vi "wformFileRead.vi"() -> ()   [LabVIEW 2014]
uses:
  <vilib>/Waveform/WDTFileIO.llb/Read Waveforms from File.vi
  <vilib>/Waveform/WDTFileIO.llb/Read Waveform from File.vi
panel:
  out "Loaded Waveform Graph":waveform(dbl)[](graph)
  out "Waveform File I/O Error":errorcluster
  out "Waveform file path":path
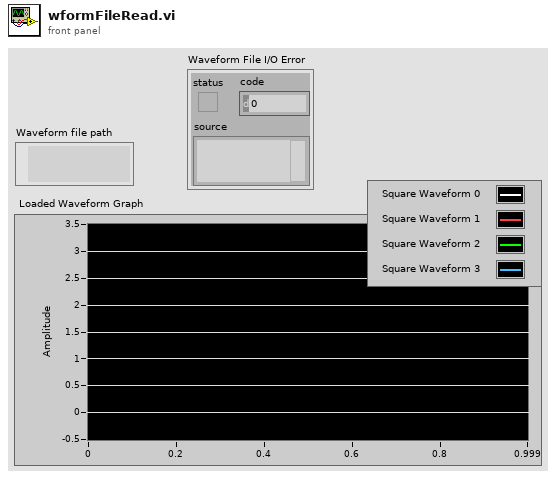
[diagram p1: front panel]
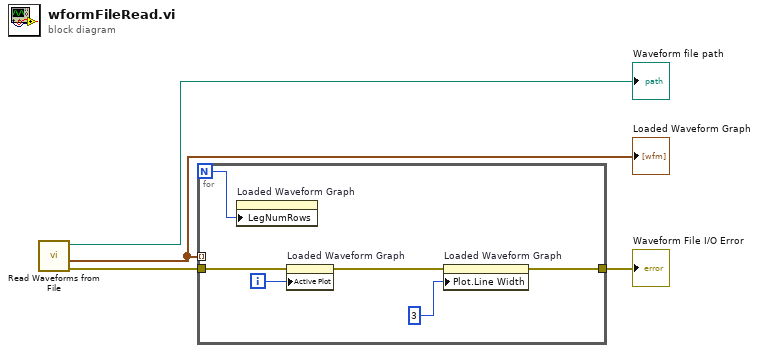
[diagram p0: block diagram]
diagram:
  n1 = call-poly "Read Waveforms from File"() -> ("error out"=w2:errorcluster, "all waveforms in record"=w3:waveform(dbl)[], "new file path (Not A Path if cancelled)"=→"Waveform file path":path)  [unwired: 6 in, 1 out]
  "Loaded Waveform Graph" <- w3
  n2 = for {
    N -> [w5]
    tunnel: w3 -> [_] mode=indexing
    tunnel: w2 -> [w8]
    tunnel: [w6] -> w1
    i -> [w9]
    n3 = property on="Loaded Waveform Graph" class="WFGraph (strict)"("LegNumRows"=w5) -> ()  [unwired: 2 in, 2 out]
    n4 = property on="Loaded Waveform Graph" class="WFGraph (strict)"(error in=w8, "Active Plot"=w9) -> (error out=w7:errorcluster)  [unwired: 1 in, 1 out]
    n5 = property on="Loaded Waveform Graph" class="WFGraph (strict)"(error in=w7, "Plot.Line Width"=u8 3) -> (error out=w6:errorcluster)  [unwired: 1 in, 1 out]
  }
  "Waveform File I/O Error" <- w1
